vi "getWeight.vi"(11 "Array":dbl[](array[numeric])) -> (3 "Weight":i32[](array[numeric]))   [LabVIEW 2014]
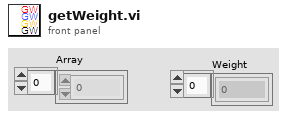
[diagram p1: front panel]
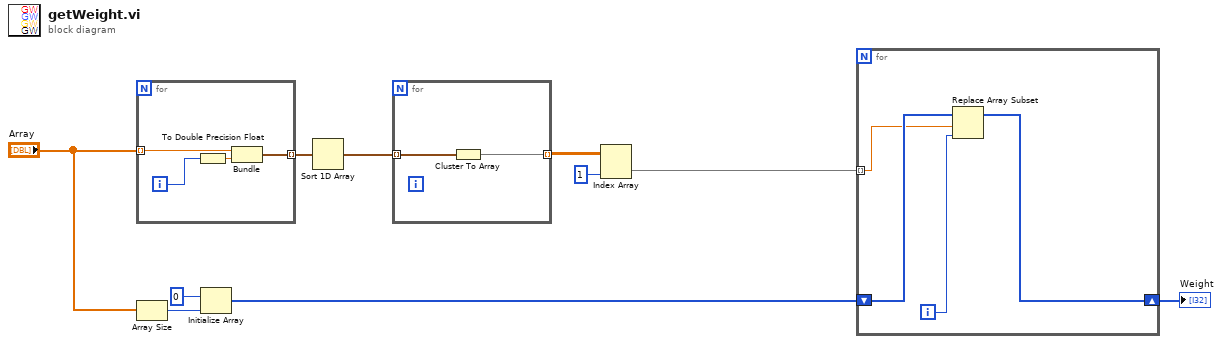
[diagram p0: block diagram]
diagram:
  n1 = for {
    tunnel: "Array" -> [w12] mode=indexing
    tunnel: [w11] -> w7 mode=indexing
    i -> [w14]
    n2 = To Double Precision Float(number=w14) -> (double precision float=w13:dbl)
    n3 = Bundle("Numeric"=w12, w13) -> (w11:cluster{"Numeric":dbl, dbl})  [unwired: 1 in]
  }
  n4 = Array Size(array="Array") -> (size(s)=w10:i32)
  n5 = Initialize Array(0 ("element"), w10) -> (w3:i32[])
  n6 = Sort 1D Array(array=w7) -> (sorted array=w6:cluster{"Numeric":dbl, dbl}[])
  n7 = for {
    tunnel: w6 -> [w16] mode=indexing
    tunnel: [w15] -> w5 mode=indexing
    n8 = Cluster To Array(cluster=w16) -> (array=w15:dbl[])
  }
  n9 = Index Array(array=w5, index (col)=1 ("index")) -> (element=w2:dbl[])  [unwired: 1 in]
  n10 = for {
    tunnel: w2 -> [w18] mode=indexing
    shift-right: [w17] -> w1
    shift-left: w3 -> [w19]
    i -> [w20]
    n11 = Replace Array Subset(array=w19, new element=w20, index=w18) -> (w17:i32[])
  }
  "Weight" <- w1
